vi "Enqueue Command.vi"(4 "ack timeout (0 ms: no ack)":i32, 6 "query notifier":refnum<notifier>, 8 "error in (no error)":errorcluster, 9 "args":variant, 10 "command":string, 11 "Queue in":refnum<queue>) -> (0 "error out":errorcluster, 1 "Ack?":bool, 3 "Queue out":refnum<queue>)   [LabVIEW 2013, in "CfgManager.Text.lvlib" / "ConfigManager.Text.lvclass"]
uses:
  ConfigManager.Text.lvclass
  payload -- cluster.ctl
  Response - cluster.ctl
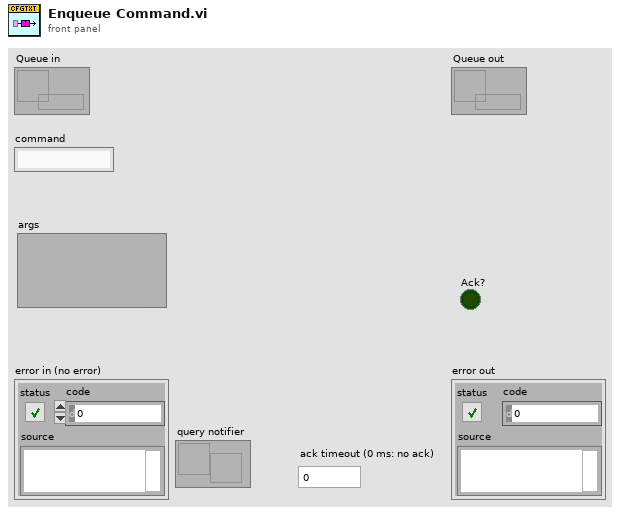
[diagram p1: front panel]
types:
  T1 = typedef "CfgManager.Text.lvlib/ConfigManager.Text.lvclass/payload -- cluster.ctl" = cluster{"command":string, "args":variant, "query":refnum<notifier>, "ack":refnum<notifier>}
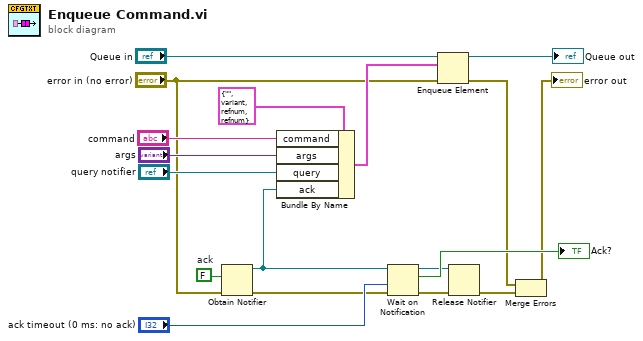
[diagram p0: block diagram]
diagram:
  w4 = FALSE  # ack
  n1 = Obtain Notifier(notification data type=w4, error in (no error)="error in (no error)") -> (notifier out=w11:refnum<notifier>, error out=w3:errorcluster)  [unwired: 2 in, 1 out]
  n2 = Bundle By Name(cluster=T1 {"command"="", "args"=variant, "query"=refnum, "ack"=refnum} ("payload"), "command"="command", "args"="args", "query"="query notifier", "ack"=w11) -> (w18:T1)
  n3 = Wait on Notification(notifier=w11, timeout in ms (-1)="ack timeout (0 ms: no ack)", error in (no error)=w3) -> (notifier out=w2:refnum<notifier>, notification=→"Ack?":bool, error out=w1:errorcluster)  [unwired: 1 in, 1 out]
  n4 = Enqueue Element(queue="Queue in", element=w18, error in (no error)="error in (no error)") -> (queue out=→"Queue out":refnum<queue>, error out=w7:errorcluster)  [unwired: 1 in, 1 out]
  n5 = Release Notifier(notifier=w2, error in (no error)=w1) -> (error out=w8:errorcluster)  [unwired: 1 in, 2 out]
  n6 = Merge Errors(w7, w8) -> (→"error out":errorcluster)
